vi "SettingsFileDialog.vi"(8 "error in (no error)":errorcluster) -> (0 "error out":errorcluster, 3 "selected path":path)   [LabVIEW 2019, in "Controller.LV.lvclass"]
uses:
  Controller.LV.lvclass
  <vilib>/Utility/sysdir.llb/System Directory Type.ctl
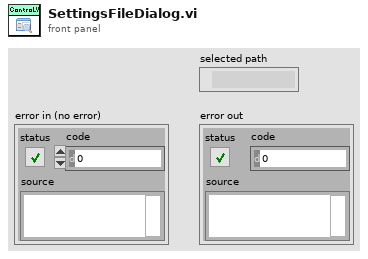
[diagram p1: front panel]
types:
  T1 = typedef "System Directory Type.ctl" = i32
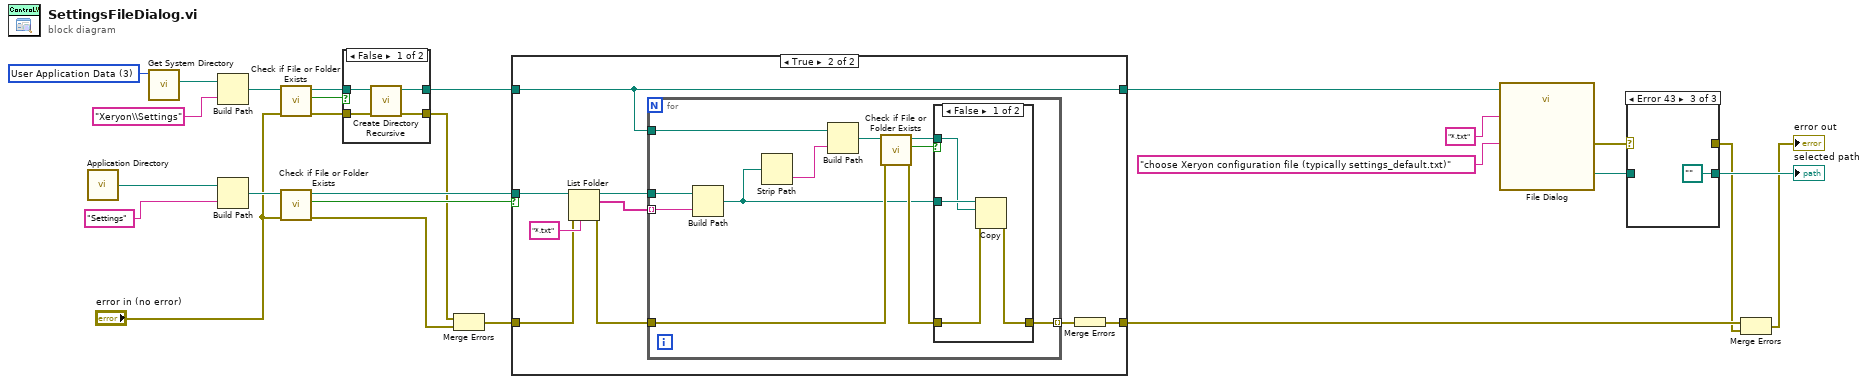
[diagram p0: block diagram]
diagram:
  w24 = T1 3 items=["User Home"=0, "User Desktop"=1, "User Documents"=2, "User Application Data"=3, "User Preferences"=4, "User Temporary"=5, "Public Documents"=6, "Public Application Data"=7, "Public Preferences"=8, "Public Cache"=13, "System Core Libraries"=9, "System Installed Libraries"=10, "Application Files"=11, "Boot Volume Root"=12] ("system directory type")
  n1 = call <vilib>:"Application Directory.vi"() -> ("Application Directory"=w21:path)
  n2 = call <vilib>:"Get System Directory.vi"("system directory type"=w24) -> ("system directory"=w23:path)  [unwired: 10 in]
  n3 = Build Path(base path=w23, name or relative path="Xeryon\\Settings") -> (appended path=w15:path)
  n4 = Build Path(base path=w21, name or relative path="Settings") -> (appended path=w18:path)
  n5 = call <vilib>:"Check if File or Folder Exists.vi"("error in (no error)"="error in (no error)", "path"=w15) -> ("error out"=w9:errorcluster, "file or folder exists?"=w14:bool, "dup path"=w12:path)  [unwired: 7 in]
  n6 = call <vilib>:"Check if File or Folder Exists.vi"("error in (no error)"="error in (no error)", "path"=w18) -> ("error out"=w5:errorcluster, "file or folder exists?"=w16:bool, "dup path"=w17:path)  [unwired: 7 in]
  n7 = case shown="False" w14 {
    tunnel: [w29 w32] -> w13
    tunnel: w12 -> [w30 w32]
    tunnel: w9 -> [w28 w31]
    tunnel: [w27 w31] -> w7
    frame False {
      n8 = call <vilib>:"Create Directory Recursive.vi"("error in (no error)"=w28, "directory"=w30) -> ("error out"=w27:errorcluster, "directory copy"=w29:path)  [unwired: 3 in, 1 out]
    }
    frame True {
    }
  }
  n9 = Merge Errors(w7, w5) -> (w6:errorcluster)
  n10 = case shown="True" w16 {
    tunnel: w13 -> [w34 w35]
    tunnel: [w34 w35] -> w19
    tunnel: w17 -> [_ w42]
    tunnel: [w33 w39] -> w3
    tunnel: w6 -> [w33 w40]
    frame False {
    }
    frame True {
      n11 = List Folder(path=w42, pattern="*.txt", error in=w40) -> (path out=w37:path, filenames=w36:string[], error out=w38:errorcluster)  [unwired: 1 in, 1 out]
      n12 = for {
        tunnel: w35 -> [w50]
        tunnel: w38 -> [w49]
        tunnel: [w47] -> w41 mode=indexing
        tunnel: w37 -> [w46]
        tunnel: w36 -> [w44] mode=indexing
        n13 = Build Path(base path=w46, name or relative path=w44) -> (appended path=w45:path)
        n14 = Strip Path(path=w45) -> (name=w54:string)  [unwired: 1 out]
        n15 = Build Path(base path=w50, name or relative path=w54) -> (appended path=w52:path)
        n16 = call <vilib>:"Check if File or Folder Exists.vi"("error in (no error)"=w49, "path"=w52) -> ("error out"=w48:errorcluster, "file or folder exists?"=w53:bool, "dup path"=w51:path)  [unwired: 7 in]
        n17 = case shown="False" w53 {
          tunnel: w51 -> [w57 _]
          tunnel: w45 -> [w58 _]
          tunnel: w48 -> [w56 w59]
          tunnel: [w55 w59] -> w47
          frame False {
            n18 = Copy(8:w56, 10:w57, 11:w58) -> (0:w55:errorcluster)  [unwired: 2 in, 2 out]
          }
          frame True {
          }
        }
      }
      n19 = Merge Errors(w41) -> (w39:errorcluster)
    }
  }
  n20 = call "File Dialog"("start path"=w19, "prompt"="choose Xeryon configuration file (typically settings_default.txt)", "pattern (all files)"="*.txt") -> ("selected path"=w10:path, "error out"=w4:errorcluster)  [unwired: 9 in, 2 out]
  n21 = case shown="Error 43" w4 {
    selector: w4 -> [w61 w63 _]
    tunnel: [w61 w63 _] -> w2
    tunnel: [w60 w62 path "" ("selected path")] -> w11
    tunnel: w10 -> [w60 w62 _]
    frame No Error {
    }
    frame Default {
    }
    frame Error {
    }
  }
  "selected path" <- w11
  n22 = Merge Errors(w3, w2) -> (→"error out":errorcluster)
